vi "Error站_SetDataUnlock.vi"(0 "ref in":T2, 1 "Lock ref in":T1, 2 "Data in":T3, 3 "error in":errorcluster) -> (6 "ref out":T2, 9 "error out":errorcluster)   [LabVIEW 2015]
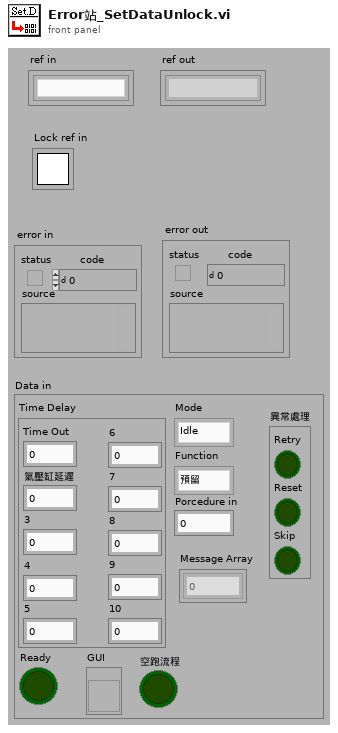
[diagram p1: front panel]
types:
  T1 = typedef "Semaphore RefNum" = refnum<k1>
  T2 = typedef "Error站_ref.ctl" = refnum<k1>
  T3 = typedef "Error站_Data.ctl" = cluster{"GUI":refnum<vi>, "Ready":bool, "Mode":T4, "Function":T5, "Porcedure in":u8, "Time Delay":cluster{"Time Out":dbl, "氣壓缸延遲":dbl, "3":dbl, "4":dbl, "5":dbl, "6":dbl, "7":dbl, "8":dbl, "9":dbl, "10":dbl}, "空跑流程":bool, "異常處理":cluster{"Retry":bool, "Reset":bool, "Skip":bool}, "Message Array":i32[]}
  T4 = typedef "Error站_Mode.ctl" = enum8{"Idle", "Run", "Pause", "Err"}
  T5 = typedef "Error站_Function.ctl" = enum8{"預留"}
  T6 = enum16{"OpenReference", "CloseReference", "Get Data", "Set Data", "Set Flag"}
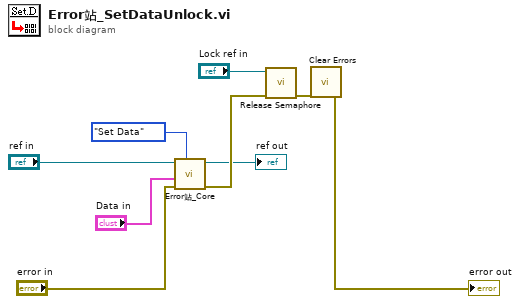
[diagram p0: block diagram]
diagram:
  n1 = call "Error站_Core.vi"("Function"=T6."Set Data", "error in"="error in", "Data in"="Data in", "ref in"="ref in") -> ("error out"=w9:errorcluster, "ref out"=→"ref out":T2)  [unwired: 4 in, 2 out]
  n2 = call <vilib>:"Release Semaphore.vi"("error in (no error)"=w9, "semaphore"="Lock ref in") -> ("error out"=w5:errorcluster)  [unwired: 4 in, 1 out]
  n3 = call <vilib>:"Clear Errors.vi"("error in (no error)"=w5) -> ("error out"=→"error out":errorcluster)  [unwired: 5 in, 1 out]
